vi "Write Roles.vi"(8 "error in (no error)":errorcluster, 10 "Roles":T1, 11 "TableWithStrikerPlay in":refnum<class "TableWithStrikerPlay.lvclass">) -> (0 "error out":errorcluster, 3 "TableWithStrikerPlay out":refnum<class "TableWithStrikerPlay.lvclass">)   [LabVIEW 2023, in "TableWithStrikerPlay.lvclass"]
uses:
  TableWithStrikerPlay.lvclass
  TableFinalizerRole_class/TableFinalizerRole.lvclass
  TablerRole_class/TablerRole.lvclass
  PassObserverRole_class/PassObserverRole.lvclass
  TableWithStrikerPlay.lvclass/TableWithStrikerPlay.ctl
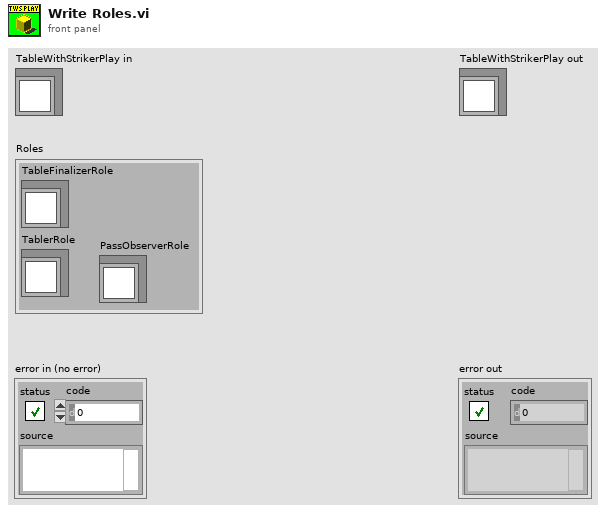
[diagram p1: front panel]
types:
  T1 = cluster{"TableFinalizerRole":refnum<class "TableFinalizerRole.lvclass">, "TablerRole":refnum<class "TablerRole.lvclass">, "PassObserverRole":refnum<class "PassObserverRole.lvclass">}
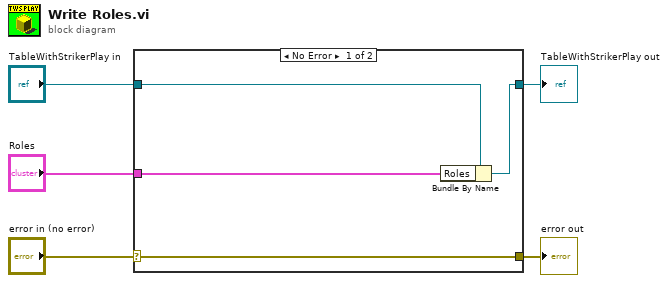
[diagram p0: block diagram]
diagram:
  n1 = case shown="No Error" "error in (no error)" {
    selector: "error in (no error)" -> [w9 w10]
    tunnel: [w9 w10] -> w4
    tunnel: [w7 w11] -> w2
    tunnel: "TableWithStrikerPlay in" -> [w8 w11]
    tunnel: "Roles" -> [w6 _]
    frame No Error {
      n2 = Bundle By Name(cluster=w8, "Roles"=w6) -> (w7:refnum<class "TableWithStrikerPlay.lvclass">)
    }
    frame Error {
    }
  }
  "error out" <- w4
  "TableWithStrikerPlay out" <- w2
